vi "Write and Read Multiple Registers Request.vi"(4 "quantity to read":u16, 6 "read starting address":u16, 8 "error in (no error)":errorcluster, 9 "write":u16[](array[numeric]), 10 "write starting address":u16) -> (0 "error out":errorcluster, 2 "Modbus data unit out":refnum<class "Modbus Data Unit (PDU).lvclass">)   [LabVIEW 2020, in "SubVIs.lvlib" / "Master Function Definition.lvlib"]
doc: "This VI forms a modbus data unit for simultaneously reading and writing multiple registers."
uses:
  <vilib>/Modbus/subvis/Data and Functions/Master Function Definition/Master Function Definition.lvlib
  <vilib>/Modbus/subvis/Modbus Data Unit (PDU)/Modbus Data Unit (PDU).lvclass
  <vilib>/Modbus/subvis/Modbus Data Unit (PDU)/Modbus Data Unit (PDU).lvclass/Modbus Data Unit (PDU).ctl
  <vilib>/Modbus/subvis/SubVIs.lvlib
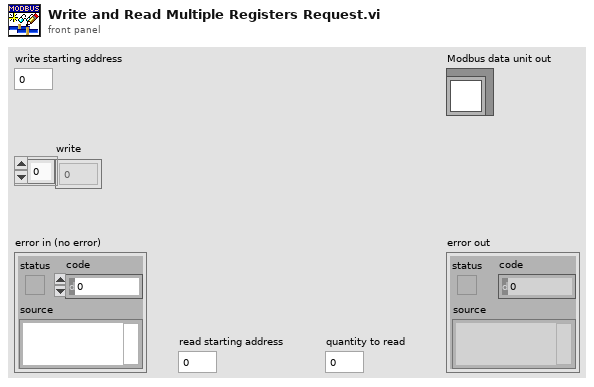
[diagram p1: front panel]
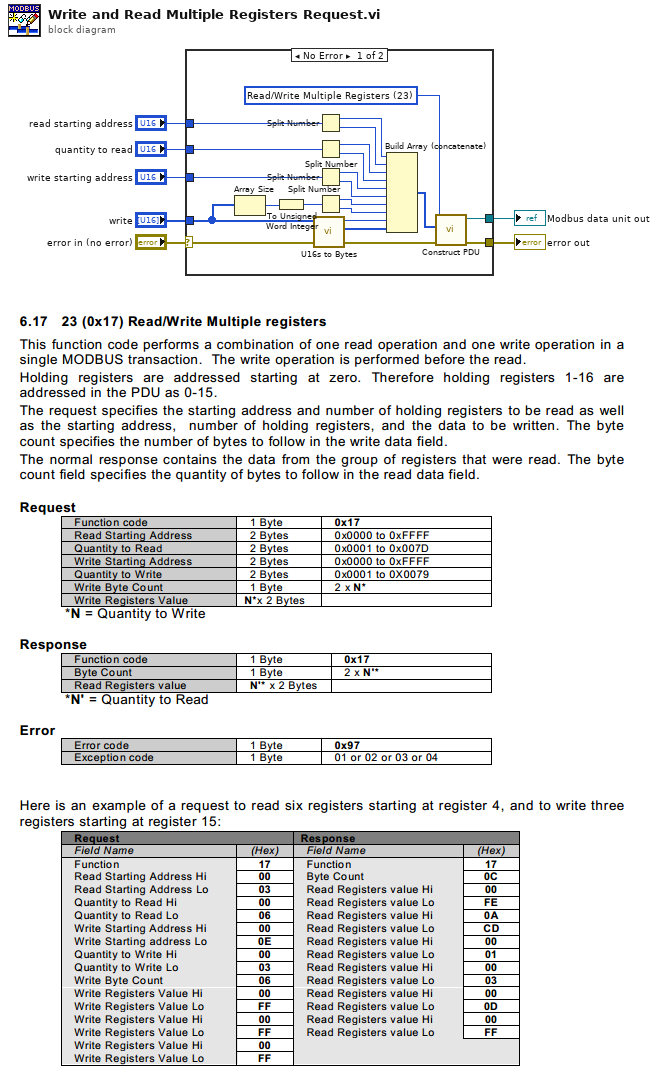
[diagram p0: block diagram]
diagram:
  n1 = case shown="No Error" "error in (no error)" {
    selector: "error in (no error)" -> [w8 w29]
    tunnel: [w28 w29] -> w7
    tunnel: "write starting address" -> [w27 _]
    tunnel: [w26 _] -> w5
    tunnel: "write" -> [w19 _]
    tunnel: "read starting address" -> [w14 _]
    tunnel: "quantity to read" -> [w13 _]
    frame No Error {
      w20 = u8 23 items=["Read Discrete Inputs"=2, "Read Coils"=1, "Write Single Coil"=5, "Write Multiple Coils"=15, "Read Input Register"=4, "Read Holding Registers"=3, "Write Single Register"=6, "Write Multiple Registers"=16, "Read/Write Multiple Registers"=23, "Mask Write Register"=22, "Read FIFO Queue"=24, "Read File Record"=20, "Write File Record"=21, "Read Exception Status"=7, "Diagnostic"=8, "Get Com Event Counter"=11, "Get Com Event Log"=12, "Report Slave ID"=17, "Read Device Identification"=43] ("Function")
      n2 = Array Size(array=w19) -> (size(s)=w18:i32)
      n3 = To Unsigned Word Integer(number=w18) -> (unsigned 16bit integer=w17:u16)
      n4 = call <vilib>:"U16s to Bytes.vi"("registers"=w19) -> ("bytes"=w15:u8[], "count"=w16:u8)  [unwired: 9 in]
      n5 = Split Number(x=w14) -> (hi(x)=w9:u8, lo(x)=w10:u8)
      n6 = Split Number(x=w13) -> (hi(x)=w11:u8, lo(x)=w12:u8)
      n7 = Split Number(x=w27) -> (hi(x)=w22:u8, lo(x)=w23:u8)
      n8 = Split Number(x=w17) -> (hi(x)=w24:u8, lo(x)=w25:u8)
      n9 = Build Array (concatenate)(w9, w10, w11, w12, w22, w23, w24, w25, w16, w15) -> (w21:u8[])
      n10 = call <vilib>:"Construct PDU.vi"("error in (no error)"=w8, "data"=w21, "function"=w20) -> ("error out"=w28:errorcluster, "Modbus data unit out"=w26:refnum<class "Modbus Data Unit (PDU).lvclass">)  [unwired: 7 in]
    }
    frame Error {
    }
  }
  "error out" <- w7
  "Modbus data unit out" <- w5
